vi "Circle Func.vi"(10 "Y In":dbl[](array[numeric]), 11 "X In":dbl[](array[numeric])) -> (1 "Z":dbl[][](array[numeric]), 2 "Y Out":dbl[](array[numeric]), 3 "X Out":dbl[](array[numeric]))   [LabVIEW 2023]
doc: "Implements a Circle Function."
uses:
  <vilib>/gmath/interp.llb/Create Mesh Grid (2D) (x,y arrays).vi
  <vilib>/gmath/NI_Gmath.lvlib
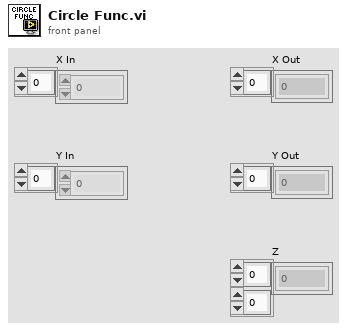
[diagram p1: front panel]
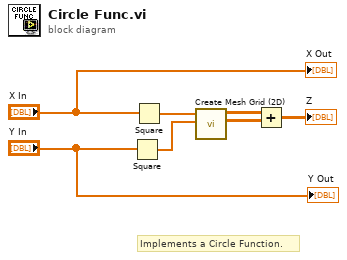
[diagram p0: block diagram]
diagram:
  # "Implements a Circle Function."
  n1 = Square(x="Y In") -> (x^2=w4:dbl[])
  n2 = Square(x="X In") -> (x^2=w5:dbl[])
  n3 = call-poly <vilib>:"Create Mesh Grid (2D).vi"("y domain"=w4, "x domain"=w5) -> ("Y"=w6:dbl[][], "X"=w7:dbl[][])  [unwired: 7 in, 1 out]
  n4 = Add(x=w7, y=w6) -> (x+y=→"Z":dbl[][])
  "X Out" <- "X In"
  "Y Out" <- "Y In"
